vi "read_settings.vi"(3 "error in":errorcluster, 5 "Path":path) -> (0 "error out":errorcluster, 1 "Pathout":path, 2 "settings_clus_file":T1={"CollectionInfoArray"=[{"Type"="Signal and Background", "LaserWave1"=249.7, "Shutter1"=TRUE, "LaserWave2"=0.0, "Shutter2"=FALSE, "FileEnd"="_SignalBack", "Collect"=TRUE}], "Delay scan"=FALSE, "channel enabled"=FALSE, "accurate scan"=FALSE, "update"=FALSE, "collection time"=0})   [LabVIEW 2019]
doc: "Reads in an xml settings file to a settings cluster"
uses:
  Type defs/settings_file_ctrl.ctl
  Type defs/FileAcq_v1_Ctrl.ctl
  <vilib>/NI/GXML/_subVIs/GXML SearchParser/Search Parser.vi
  <vilib>/NI/GXML/GXML.lvlib
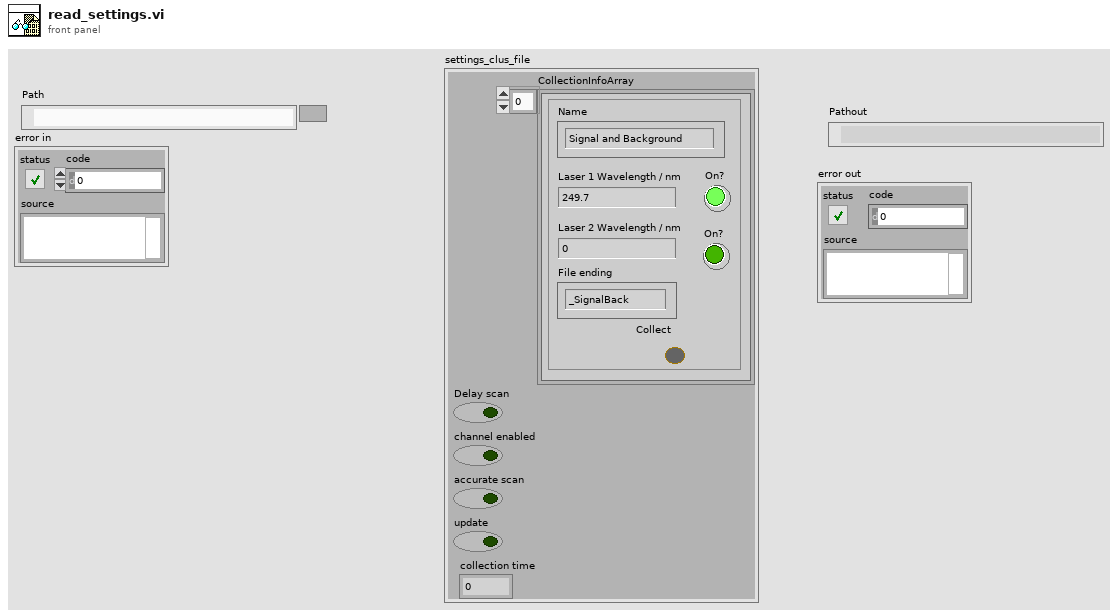
[diagram p1: front panel]
types:
  T1 = typedef "settings_file_ctrl.ctl" = cluster{"CollectionInfoArray":T2[], "Delay scan":bool, "channel enabled":bool, "accurate scan":bool, "update":bool, "collection time":i32}
  T2 = typedef "FileAcq_v1_Ctrl.ctl" = cluster{"Type":string, "LaserWave1":dbl, "Shutter1":bool, "LaserWave2":dbl, "Shutter2":bool, "FileEnd":string, "Collect":bool}
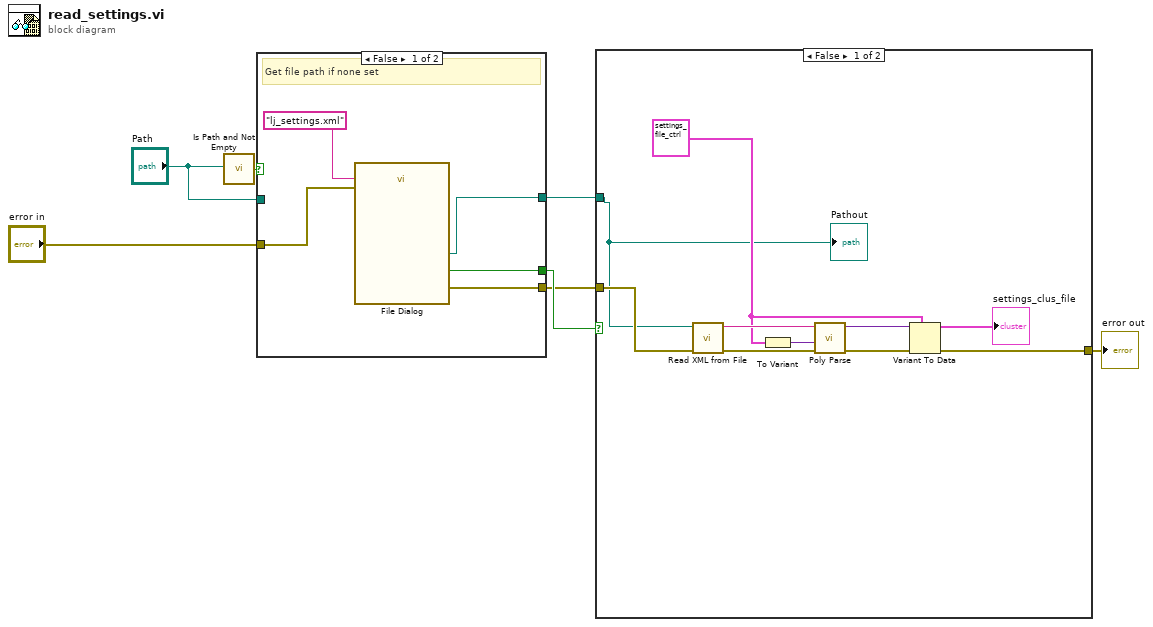
[diagram p0: block diagram]
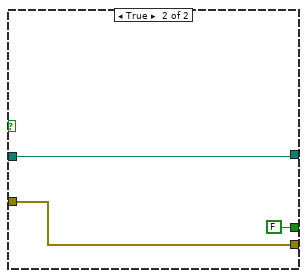
[diagram p3: hidden frame]
diagram:
  n1 = call <vilib>:"Is Path and Not Empty.vi"("path"="Path") -> ("Is Path and Not Empty?"=w7:bool)  [unwired: 4 in]
  n2 = case shown="False" w7 {
    tunnel: [w10 w15] -> w4
    tunnel: "Path" -> [_ w15]
    tunnel: [w12 w14] -> w2
    tunnel: "error in" -> [w11 w14]
    tunnel: [w9 FALSE ("cancelled")] -> w3
    frame False {
      # "Get file path if none set"
      n3 = call "File Dialog"("default name"="lj_settings.xml", "error in"=w11) -> ("selected path"=w10:path, "cancelled"=w9:bool, "error out"=w12:errorcluster)  [unwired: 10 in, 1 out]
    }
    frame True {
    }
  }
  n4 = case shown="False" w3 {
    tunnel: w4 -> [w16 _]
    tunnel: w2 -> [w25 w26]
    tunnel: [w17 w26] -> w1
    frame False {
      w19 = T1 {"CollectionInfoArray"=[{"Type"="Signal and Background", "LaserWave1"=249.7, "Shutter1"=TRUE, "LaserWave2"=0.0, "Shutter2"=FALSE, "FileEnd"="_SignalBack", "Collect"=TRUE}], "Delay scan"=FALSE, "channel enabled"=FALSE, "accurate scan"=FALSE, "update"=FALSE, "collection time"=0} ("settings_clus_file")
      n5 = call <vilib>:"Read XML from File.vi"("error in"=w25, "XML File Path"=w16) -> ("error out"=w24:errorcluster, "XML String Out"=w22:string)  [unwired: 8 in]
      n6 = To Variant(anything=w19) -> (Variant=w23:variant)
      n7 = call-poly <vilib>:"Poly Parse.vi"("error in"=w24, "TypeDesc"=w23, "XML String In"=w22) -> ("error out"=w21:errorcluster, "Parsed Data"=w20:variant)  [unwired: 7 in]
      n8 = Variant To Data(error in=w21, type=w19, Variant=w20) -> (data=→"settings_clus_file":T1, error out=w17:errorcluster)
      "Pathout" <- w16
    }
    frame True {
    }
  }
  "error out" <- w1
